vi "Func-엑셀 데이터를 그래프로 출력.vi"() -> ()   [LabVIEW 2015] (continued)
-40\t-40.02\t-26.852\n-40\t-40.02\t-26.858\n-40\t-40\t-26.864\n-40\t-40\t-26.866\n-40\t-40\t-26.87\n-40\t-40\t-26.875\n-40\t-40\t-26.878\n-40\t-40\t-26.884\n-40\t-40\t-26.888\n-40\t-40\t-26.889\n-40\t-40\t-26.893\n-40\t-40\t-26.896\n-40\t-40\t-26.899\n-40\t-40\t-26.902\n-40\t-40\t-26.903\n-40\t-40\t-26.909\n-40\t-40\t-26.915\n-40\t-40\t-26.918\n-40\t-40\t-26.925\n-40\t-40\t-26.93\n-40\t-40\t-26.935\n-40\t-40\t-26.936\n-40\t-40\t-26.938\n-40\t-40\t-26.943\n-40\t-40\t-26.944\n-40\t-40\t-26.948\n-40\t-40\t-26.952\n-40\t-40\t-26.958\n-40\t-40\t-26.965\n-40\t-40\t-26.968\n-40\t-40\t-26.972\n-40\t-40\t-26.973\n-40\t-40\t-26.979\n-40\t-40\t-26.978\n-40\t-40\t-26.982\n-40\t-40\t-26.987\n-40\t-40\t-26.992\n-40\t-40\t-27\n-40\t-40\t-27.002\n-40\t-40\t-27.007\n-40\t-40\t-27.009\n-40\t-40\t-27.012\n-40\t-40\t-27.013\n-40\t-40\t-27.022\n-40\t-40\t-27.022\n-40\t-40\t-27.027\n-40\t-40\t-27.032\n-40\t-40\t-27.035\n-40\t-40\t-27.038\n-40\t-40\t-27.037\n-40\t-40\t-27.04\n-40\t-40\t-27.042\n-40\t-40\t-27.049\n-40\t-40\t-27.05\n-40\t-40\t-27.053\n-40\t-40\t-27.059\n-40\t-40\t-27.064\n-40\t-40\t-27.07\n-40\t-40\t-27.073\n-40\t-40.02\t-27.078\n-40\t-40.02\t-27.08\n-40\t-40.02\t-27.088\n-40\t-40.02\t-27.095\n-40\t-40.02\t-27.096\n-40\t-40.02\t-27.103\n-40\t-40.02\t-27.105\n-40\t-40.02\t-27.11\n-40\t-40.02\t-27.113\n-40\t-40.02\t-27.11\n-40\t-40.02\t-27.114\n-40\t-40.02\t-27.115\n-40\t-40.02\t-27.12\n-40\t-40.02\t-27.123\n-40\t-40.02\t-27.126\n-40\t-40.02\t-27.132\n-40\t-40.02\t-27.136\n-40\t-40.02\t-27.143\n-40\t-40.02\t-27.143\n-40\t-40.02\t-27.145\n-40\t-40.02\t-27.148\n-40\t-40.02\t-27.153\n-40\t-40.02\t-27.157\n-40\t-40.02\t-27.164\n-40\t-40.02\t-27.168\n-40\t-40.02\t-27.173\n-40\t-40.02\t-27.18\n-40\t-40.02\t-27.184\n-40\t-40.02\t-27.186\n-40\t-40.02\t-27.184\n-40\t-40.02\t-27.19\n-40\t-40.02\t-27.194\n-40\t-40.02\t-27.196\n-40\t-40.02\t-27.2\n-40\t-40.02\t-27.202\n-40\t-40.02\t-27.209\n-40\t-40.02\t-27.208\n-40\t-40.02\t-27.211\n-40\t-40.02\t-27.219\n-40\t-40.02\t-27.222\n-40\t-40.02\t-27.227\n-40\t-40.02\t-27.23\n-40\t-40.02\t-27.237\n-40\t-40.02\t-27.241\n-40\t-40.02\t-27.241\n-40\t-40.02\t-27.243\n-40\t-40.02\t-27.248\n-40\t-40.02\t-27.255\n-40\t-40.02\t-27.257\n-40\t-40.02\t-27.259\n-40\t-40.02\t-27.264\n-40\t-40.02\t-27.268\n-40\t-40.02\t-27.27\n-40\t-40.02\t-27.277\n-40\t-40.02\t-27.278\n-40\t-40.02\t-27.279\n-40\t-40.02\t-27.282\n-40\t-40.02\t-27.284\n-40\t-40.02\t-27.285\n-40\t-40.02\t-27.283\n-40\t-40.02\t-27.286\n-40\t-40.02\t-27.293\n-40\t-40.02\t-27.298\n-40\t-40.02\t-27.303\n-40\t-40.02\t-27.308\n-40\t-40.02\t-27.312\n-40\t-40.02\t-27.315\n-40\t-40.02\t-27.318\n-40\t-40.02\t-27.324\n-40\t-40\t-27.327\n-40\t-40\t-27.33\n-40\t-40\t-27.335\n-40\t-40\t-27.342\n-40\t-40\t-27.344\n-40\t-40\t-27.344\n-40\t-40\t-27.349\n-40\t-40\t-27.349\n-40\t-40\t-27.355\n-40\t-40\t-27.356\n-40\t-40\t-27.361\n-40\t-40\t-27.371\n-40\t-40\t-27.373\n-40\t-40\t-27.375\n-40\t-40\t-27.382\n-40\t-40\t-27.385\n-40\t-40\t-27.388\n-40\t-40\t-27.389\n-40\t-40\t-27.393\n-40\t-40\t-27.398\n-40\t-40\t-27.397\n-40\t-40\t-27.398\n-40\t-40\t-27.401\n-40\t-40\t-27.401\n-40\t-40\t-27.404\n-40\t-40\t-27.412\n-40\t-40\t-27.414\n-40\t-40\t-27.417\n-40\t-40\t-27.421\n-40\t-40\t-27.429\n-40\t-40\t-27.431\n-40\t-40\t-27.435\n-40\t-40\t-27.439\n-40\t-40\t-27.444\n-40\t-40\t-27.443\n-40\t-40\t-27.449\n-40\t-40\t-27.451\n-40\t-40\t-27.453\n-40\t-40\t-27.453\n-40\t-40\t-27.453\n-40\t-40\t-27.456\n-40\t-40\t-27.461\n-40\t-40\t-27.461\n-40\t-40\t-27.466\n-40\t-40\t-27.473\n-40\t-40\t-27.477\n-40\t-40\t-27.481\n-40\t-40\t-27.482\n-40\t-40\t-27.488\n-40\t-40\t-27.492\n-40\t-40\t-27.497\n-40\t-40\t-27.502\n-40\t-40\t-27.504\n-40\t-40\t-27.507\n-40\t-40\t-27.507\n-40\t-40\t-27.51\n-40\t-40\t-27.515\n-40\t-40\t-27.516\n-40\t-40\t-27.524\n-40\t-40\t-27.533\n-40\t-40\t-27.538\n-40\t-40\t-27.54\n-40\t-40\t-27.539\n-40\t-40\t-27.543\n-40\t-40\t-27.546\n-40\t-40\t-27.546\n-40\t-40\t-27.548\n-40\t-40\t-27.549\n-40\t-40\t-27.553\n-40\t-40\t-27.557\n-40\t-40\t-27.557\n-40\t-40\t-27.559\n-40\t-40\t-27.562\n-40\t-40\t-27.569\n-40\t-40\t-27.572\n-40\t-40\t-27.571\n-40\t-40\t-27.579\n-40\t-40\t-27.582\n-40\t-40\t-27.586\n-40\t-40\t-27.588\n-40\t-40\t-27.591\n-40\t-40\t-27.594\n-40\t-40\t-27.595\n-40\t-40\t-27.595\n-40\t-40\t-27.599\n-40\t-40\t-27.605\n-40\t-40\t-27.607\n-40\t-40\t-27.61\n-40\t-40\t-27.613\n-40\t-40\t-27.616\n-40\t-40\t-27.619\n-40\t-40\t-27.623\n-40\t-40\t-27.627\n-40\t-40\t-27.634\n-40\t-40\t-27.64\n-40\t-40\t-27.646\n-40\t-40\t-27.647\n-40\t-40\t-27.652\n-40\t-40\t-27.654\n-40\t-40\t-27.654\n-40\t-40\t-27.655\n-40\t-40\t-27.655\n-40\t-40\t-27.658\n-40\t-40\t-27.659\n-40\t-40\t-27.663\n-40\t-40\t-27.668\n-40\t-40\t-27.674\n-40\t-40\t-27.675\n-40\t-40\t-27.678\n-40\t-40\t-27.682\n-40\t-40\t-27.687\n-40\t-40\t-27.686\n-40\t-40\t-27.689\n-40\t-40\t-27.695\n-40\t-40\t-27.698\n-40\t-40\t-27.703\n-40\t-40\t-27.705\n-40\t-40\t-27.707\n-40\t-40\t-27.712\n-40\t-40\t-27.714\n-40\t-40\t-27.715\n-40\t-40\t-27.719\n-40\t-40\t-27.721\n-40\t-40\t-27.726\n-40\t-40\t-27.729\n-40\t-40\t-27.732\n-40\t-40\t-27.734\n-40\t-40\t-27.735\n-40\t-40\t-27.734\n-40\t-40\t-27.738\n-40\t-40\t-27.739\n-40\t-40\t-27.741\n-40\t-40\t-27.746\n-40\t-40\t-27.753\n-40\t-40\t-27.758\n-40\t-40\t-27.762\n-40\t-40\t-27.762\n-40\t-40\t-27.765\n-40\t-40\t-27.769\n-40\t-40\t-27.768\n-40\t-40\t-27.769\n-40\t-40\t-27.77\n-40\t-40\t-27.777\n-40\t-40\t-27.781\n-40\t-40\t-27.781\n-40\t-40\t-27.788\n-40\t-40\t-27.793\n-40\t-40\t-27.796\n-40\t-40\t-27.8\n-40\t-40\t-27.804\n-40\t-40\t-27.807\n-40\t-40\t-27.809\n-40\t-40\t-27.81\n-40\t-40\t-27.811\n-40\t-40\t-27.815\n-40\t-40\t-27.814\n-40\t-40\t-27.816\n-40\t-40\t-27.821\n-40\t-40\t-27.825\n-40\t-40\t-27.827\n-40\t-40\t-27.831\n-40\t-40\t-27.835\n-40\t-40\t-27.837\n-40\t-40\t-27.841\n-40\t-40\t-27.843\n-40\t-40\t-27.846\n-40\t-40\t-27.85\n-40\t-40\t-27.854\n-40\t-40\t-27.858\n-40\t-40\t-27.862\n-40\t-40\t-27.864\n-40\t-40\t-27.868\n-40\t-40\t-27.871\n-40\t-40\t-27.877\n-40\t-40\t-27.878\n-40\t-40\t-27.88\n-40\t-40\t-27.883\n-40\t-40\t-27.884\n-40\t-40\t-27.885\n-40\t-40\t-27.885\n-40\t-40\t-27.888\n-40\t-40\t-27.889\n-40\t-40\t-27.891\n-40\t-40\t-27.895\n-40\t-40\t-27.902\n-40\t-40\t-27.903\n-40\t-40\t-27.905\n-40\t-40\t-27.908\n-40\t-40\t-27.909\n-40\t-40\t-27.914\n-40\t-40\t-27.914\n-40\t-40\t-27.918\n-40\t-40\t-27.918\n-40\t-40\t-27.921\n-40\t-40\t-27.927\n-40\t-40\t-27.927\n-40\t-40\t-27.933\n-40\t-40\t-27.936\n-40\t-40\t-27.939\n-40\t-40\t-27.943\n-40\t-40\t-27.943\n-40\t-40\t-27.949\n-40\t-40\t-27.955\n-40\t-40\t-27.957\n-40\t-40\t-27.962\n-40\t-40\t-27.966\n-40\t-40\t-27.966\n-40\t-40\t-27.963\n-40\t-40\t-27.963\n-40\t-40\t-27.966\n-40\t-40\t-27.968\n-40\t-40\t-27.971\n-40\t-40\t-27.975\n-40\t-40\t-27.979\n-40\t-40\t-27.981\n-40\t-40\t-27.982\n-40\t-40\t-27.983\n-40\t-40\t-27.98\n-40\t-40\t-27.983\n-40\t-40\t-27.984\n-40\t-40\t-27.989\n-40\t-40\t-27.991\n-40\t-40\t-27.997\n-40\t-40\t-28.002\n-40\t-40\t-28.004\n-40\t-40\t-28.005\n-40\t-40\t-28.006\n-40\t-40\t-28.013\n-40\t-40\t-28.016\n-40\t-40\t-28.018\n-40\t-40\t-28.021\n-40\t-40\t-28.029\n-40\t-40\t-28.032\n-40\t-40\t-28.031\n-40\t-40\t-28.034\n-40\t-40\t-28.037\n-40\t-40\t-28.043\n-40\t-40\t-28.045\n-40\t-40\t-28.045\n-40\t-40\t-28.048\n-40\t-40\t-28.049\n-40\t-40\t-28.052\n-40\t-40\t-28.055\n-40\t-40\t-28.062\n-40\t-40\t-28.065\n-40\t-40\t-28.067\n-40\t-40\t-28.074\n-40\t-40\t-28.076\n-40\t-40\t-28.075\n-40\t-40\t-28.076\n-40\t-40\t-28.078\n-40\t-40\t-28.077\n-40\t-40\t-28.081\n-40\t-40\t-28.087\n-40\t-40\t-28.087\n-40\t-40\t-28.09\n-40\t-40\t-28.095\n-40\t-40\t-28.102\n-40\t-40\t-28.103\n-40\t-40\t-28.102\n-40\t-40\t-28.104\n-40\t-40\t-28.108\n-40\t-40\t-28.108\n-40\t-40\t-28.108\n-40\t-40\t-28.108\n-40\t-40\t-28.111\n-40\t-40\t-28.117\n-40\t-40\t-28.117\n-40\t-40\t-28.119\n-40\t-40\t-28.121\n-40\t-40\t-28.125\n-40\t-40\t-28.125\n-40\t-40\t-28.127\n-40\t-40\t-28.129\n-40\t-40\t-28.134\n-40\t-40\t-28.135\n-40\t-40\t-28.139\n-40\t-40\t-28.141\n-40\t-40\t-28.143\n-40\t-40\t-28.149\n-40\t-40\t-28.153\n-40\t-40\t-28.155\n-40\t-40\t-28.157\n-40\t-40\t-28.16\n-40\t-40\t-28.164\n-40\t-40\t-28.165\n-40\t-40\t-28.17\n-40\t-40\t-28.175\n-40\t-40\t-28.18\n-40\t-40\t-28.183\n-40\t-40\t-28.182\n-40\t-40\t-28.186\n-40\t-40\t-28.182\n-40\t-40\t-28.182\n-40\t-40\t-28.184\n-40\t-40\t-28.184\n-40\t-40\t-28.19\n-40\t-40\t-28.194\n-40\t-40\t-28.198\n-40\t-40\t-28.203\n-40\t-40\t-28.205\n-40\t-40\t-28.208\n-40\t-40\t-28.209\n-40\t-40\t-28.21\n-40\t-40\t-28.212\n-40\t-40\t-28.212\n-40\t-40\t-28.217\n-40\t-40\t-28.221\n-40\t-40\t-28.223\n-40\t-40\t-28.225\n-40\t-40\t-28.223\n-40\t-40\t-28.228\n-40\t-40\t-28.23\n-40\t-40\t-28.233\n-40\t-40\t-28.233\n-40\t-40\t-28.236\n-40\t-40\t-28.239\n-40\t-40\t-28.237\n-40\t-40\t-28.239\n-40\t-40\t-28.24\n-40\t-40\t-28.244\n-40\t-40\t-28.245\n-40\t-40\t-28.25\n-40\t-40\t-28.255\n-40\t-40\t-28.258\n-40\t-40\t-28.259\n-40\t-40\t-28.261\n-40\t-40\t-28.263\n-40\t-40\t-28.265\n-40\t-40\t-28.264\n-40\t-40\t-28.261\n-40\t-40\t-28.263\n-40\t-40\t-28.269\n-40\t-40\t-28.273\n-40\t-40\t-28.273\n-40\t-40\t-28.277\n-40\t-40\t-28.284\n-40\t-40\t-28.29\n-40\t-40\t-28.288\n-40\t-40\t-28.291\n-40\t-40\t-28.295\n-40\t-40\t-28.298\n-40\t-40\t-28.3\n-40\t-40\t-28.298\n-40\t-40\t-28.302\n-40\t-40\t-28.307\n-40\t-40\t-28.308\n-40\t-40\t-28.313\n-40\t-40\t-28.314\n-40\t-40\t-28.318\n-40\t-40\t-28.321\n-40\t-40\t-28.319\n-40\t-40\t-28.322\n-40\t-40\t-28.318\n-40\t-40\t-28.322\n-40\t-40\t-28.324\n-40\t-40\t-28.323\n-40\t-40\t-28.329\n-40\t-40\t-28.334\n-40\t-40\t-28.337\n-40\t-40\t-28.343\n-40\t-40\t-28.343\n-40\t-40\t-28.347\n-40\t-40\t-28.351\n-40\t-40\t-28.348\n-40\t-40\t-28.352\n-40\t-40\t-28.354\n-40\t-40\t-28.355\n-40\t-40\t-28.356\n-40\t-40\t-28.355\n-40\t-40\t-28.36\n-40\t-40\t-28.36\n-40\t-40\t-28.357\n-40\t-40\t-28.362\n-40\t-40\t-28.365\n-40\t-40\t-28.369\n-40\t-40\t-28.371\n-40\t-40\t-28.373\n-40\t-40\t-28.38\n-40\t-40\t-28.381\n-40\t-40\t-28.384\n-40\t-40\t-28.384\n-40\t-40\t-28.388\n-40\t-40\t-28.391\n-40\t-40\t-28.391\n-40\t-40\t-28.391\n-40\t-40\t-28.394\n-40\t-40\t-28.395\n-40\t-40\t-28.394\n-40\t-40\t-28.398\n-40\t-40\t-28.403\n-40\t-40\t-28.404\n-40\t-40\t-28.406\n-40\t-40\t-28.409\n-40\t-40\t-28.413\n-40\t-40\t-28.411\n-40\t-40\t-28.411\n-40\t-40\t-28.412\n-40\t-40\t-28.417\n-40\t-40\t-28.418\n-40\t-40\t-28.42\n-40\t-40\t-28.425\n-40\t-40\t-28.43\n-40\t-40\t-28.434\n-40\t-40\t-28.435\n-40\t-40\t-28.436\n-40\t-40\t-28.436\n-40\t-40\t-28.44\n-40\t-40\t-28.44\n-40\t-40\t-28.445\n-40\t-40\t-28.446\n-40\t-40\t-28.449\n-40\t-40\t-28.451\n-40\t-40\t-28.449\n-40\t-40\t-28.45\n-40\t-40\t-28.45\n-40\t-40\t-28.452\n-40\t-40\t-28.451\n-40\t-40\t-28.457\n-40\t-40\t-28.46\n-40\t-40\t-28.46\n-40\t-40\t-28.459\n-40\t-40\t-28.464\n-40\t-40\t-28.469\n-40\t-40\t-28.467\n-40\t-40\t-28.471\n-40\t-40\t-28.474\n-40\t-40\t-28.479\n-40\t-40\t-28.478\n-40\t-40\t-28.478\n-40\t-40.02\t-28.479\n-40\t-40.02\t-28.481\n-40\t-40.02\t-28.486\n-40\t-40\t-28.489\n-40\t-40.02\t-28.49\n-40\t-40\t-28.491\n-40\t-40\t-28.493\n-40\t-40\t-28.492\n-40\t-40\t-28.492\n-40\t-40\t-28.488\n-40\t-40\t-28.497\n-40\t-40\t-28.503\n-40\t-40\t-28.502\n-40\t-40\t-28.507\n-40\t-40\t-28.513\n-40\t-40.02\t-28.519\n-40\t-40.02\t-28.517\n-40\t-40.02\t-28.516\n-40\t-40.02\t-28.522\n-40\t-40.02\t-28.526\n-40\t-40\t-28.524\n-40\t-40\t-28.527\n-40\t-40\t-28.534\n-40\t-40\t-28.535\n-40\t-40.02\t-28.536\n-40\t-40.02\t-28.538\n-40\t-40.02\t-28.54\n-40\t-40.02\t-28.539\n-40\t-40.02\t-28.539\n-40\t-40.02\t-28.54\n-40\t-40.02\t-28.543\n-40\t-40.02\t-28.546\n-40\t-40.02\t-28.547\n-40\t-40.02\t-28.549\n-40\t-40.02\t-28.549\n-40\t-40.02\t-28.553\n-40\t-40.02\t-28.554\n-40\t-40.02\t-28.555\n-40\t-40.02\t-28.559\n-40\t-40.02\t-28.564\n-40\t-40.02\t-28.565\n-40\t-40\t-28.564\n-40\t-40\t-28.565\n-40\t-40\t-28.567\n-40\t-40\t-28.567\n-40\t-40\t-28.565\n-40\t-40\t-28.566\n-40\t-40\t-28.569\n-40\t-40\t-28.57\n-40\t-40\t-28.574\n-40\t-40.02\t-28.577\n-40\t-40\t-28.579\n-40\t-40\t-28.584\n-40\t-40\t-28.586\n-40\t-40\t-28.589\n-40\t-40\t-28.59\n-40\t-40\t-28.589\n-40\t-40\t-28.591\n-40\t-40\t-28.594\n-40\t-40\t-28.595\n-40\t-40\t-28.595\n-40\t-40\t-28.598\n-40\t-40\t-28.599\n-40\t-40\t-28.601\n-40\t-40\t-28.607\n-40\t-40\t-28.609\n-40\t-40\t-28.609\n-40\t-40\t-28.613\n-40\t-40\t-28.615\n-40\t-40\t-28.616\n-40\t-40\t-28.613\n-40\t-40\t-28.615\n-40\t-40\t-28.619\n-40\t-40\t-28.618\n-40\t-40\t-28.621\n-40\t-40\t-28.623\n-40\t-40.02\t-28.626\n-40\t-40\t-28.628\n-40\t-40\t-28.632\n-40\t-40\t-28.635\n-40\t-40\t-28.636\n-40\t-40\t-28.639\n-40\t-40\t-28.638\n-40\t-40\t-28.639\n-40\t-40\t-28.639\n-40\t-40\t-28.64\n-40\t-40\t-28.641\n-40\t-40\t-28.643\n-40\t-40\t-28.649\n-40\t-40\t-28.651\n-40\t-40\t-28.65\n-40\t-40\t-28.654\n-40\t-40\t-28.655\n-40\t-40\t-28.656\n-40\t-40\t-28.658\n-40\t-40\t-28.659\n-40\t-40\t-28.659\n-40\t-40\t-28.661\n-40\t-40\t-28.664\n-40\t-40\t-28.666\n-40\t-40\t-28.668\n-40\t-40\t-28.671\n-40\t-40\t-28.673\n-40\t-40\t-28.679\n-40\t-40\t-28.68\n-40\t-40\t-28.682\n-40\t-40\t-28.683\n-40\t-40\t-28.684\n-40\t-40\t-28.69\n-40\t-40\t-28.69\n-40\t-40\t-28.69\n-40\t-40\t-28.696\n-40\t-40\t-28.7\n-40\t-40\t-28.702\n-40\t-40\t-28.701\n-40\t-40\t-28.703\n-40\t-40\t-28.706\n-40\t-40\t-28.706\n-40\t-40\t-28.703\n-40\t-40\t-28.704\n-40\t-40\t-28.707\n-40\t-40\t-28.71\n-40\t-40\t-28.71\n-40\t-40\t-28.71\n-40\t-40\t-28.712\n-40\t-40\t-28.712\n-40\t-40\t-28.712\n-40\t-40\t-28.71\n-40\t-40\t-28.714\n-40\t-40\t-28.717\n-40\t-40\t-28.719\n-40\t-40\t-28.721\n-40\t-40\t-28.726\n-40\t-40\t-28.727\n-40\t-40\t-28.728\n-40\t-40\t-28.731\n-40\t-40\t-28.736\n-40\t-40\t-28.736\n-40\t-40\t-28.734\n-40\t-40\t-28.739\n-40\t-40\t-28.741\n-40\t-40\t-28.741\n-40\t-40\t-28.739\n-40\t-40\t-28.74\n-40\t-40\t-28.743\n-40\t-40\t-28.746\n-40\t-40\t-28.747\n-40\t-40\t-28.746\n-40\t-40\t-28.751\n-40\t-40\t-28.754\n-40\t-40\t-28.755\n-40\t-40\t-28.761\n-40\t-40\t-28.762\n-40\t-40\t-28.762\n-40\t-40\t-28.761\n-40\t-40\t-28.763\n-40\t-40\t-28.764\n-40\t-40\t-28.764\n-40\t-40\t-28.765\n-40\t-40\t-28.773\n-40\t-40\t-28.775\n-40\t-40\t-28.777\n-40\t-40\t-28.783\n-40\t-40\t-28.779\n-40\t-40\t-28.782\n-40\t-40\t-28.781\n-40\t-40\t-28.783\n-40\t-40\t-28.783\n-40\t-40\t-28.782\n-40\t-40\t-28.786\n-40\t-40\t-28.786\n-40\t-40\t-28.79\n-40\t-40\t-28.79\n-40\t-40\t-28.791\n-40\t-40\t-28.798\n-40\t-40\t-28.799\n-40\t-40\t-28.8\n-40\t-40\t-28.801\n-40\t-40\t-28.802\n-40\t-40\t-28.804\n-40\t-40\t-28.804\n-40\t-40\t-28.807\n-40\t-40\t-28.805\n-40\t-40\t-28.809\n-40\t-40\t-28.811\n-40\t-40\t-28.811\n-40\t-40\t-28.814\n-40\t-40\t-28.812\n-40\t-40\t-28.819\n-40\t-40\t-28.821\n-40\t-40\t-28.821\n-40\t-40\t-28.824\n-40\t-40\t-28.825\n-40\t-40\t-28.83\n-40\t-40\t-28.825\n-40\t-40\t-28.829\n-40\t-40\t-28.833\n-40\t-40\t-28.834\n-40\t-40\t-28.834\n-40\t-40\t-28.832\n-40\t-40\t-28.836\n-40\t-40\t-28.834\n-40\t-40\t-28.838\n-40\t-40\t-28.841\n-40\t-40\t-28.844\n-40\t-40\t-28.847\n-40\t-40\t-28.85\n-40\t-40\t-28.851\n-40\t-40\t-28.851\n-40\t-40\t-28.852\n-40\t-40\t-28.852\n-40\t-40\t-28.852\n-40\t-40\t-28.855\n-40\t-40\t-28.86\n-40\t-40\t-28.863\n-40\t-40\t-28.866\n-40\t-40\t-28.869\n-40\t-40\t-28.871\n-40\t-40\t-28.872\n-40\t-40\t-28.872\n-40\t-40\t-28.871\n-40\t-40\t-28.872\n-40\t-40\t-28.873\n-40\t-40\t-28.873\n-40\t-40\t-28.873\n-40\t-40\t-28.874\n-40\t-40\t-28.875\n-40\t-40\t-28.875\n-40\t-40\t-28.879\n-40\t-40\t-28.885\n-40\t-40\t-28.884\n-40\t-40\t-28.886\n-40\t-40\t-28.891\n-40\t-40\t-28.893\n-40\t-40\t-28.893\n-40\t-40\t-28.891\n-40\t-40\t-28.893\n-40\t-40\t-28.896\n-40\t-40\t-28.895\n-40\t-40\t-28.898\n-40\t-40\t-28.9\n-40\t-40\t-28.9\n-40\t-40\t-28.902\n-40\t-40\t-28.904\n-40\t-40\t-28.906\n-40\t-40\t-28.907\n-40\t-40\t-28.908\n-40\t-40\t-28.909\n-40\t-40\t-28.908\n-40\t-40\t-28.911\n-40\t-40\t-28.911\n-40\t-40\t-28.914\n-40\t-40\t-28.913\n-40\t-40\t-28.916\n-40\t-40\t-28.917\n-40\t-40\t-28.915\n-40\t-40\t-28.915\n-40\t-40\t-28.913\n-40\t-40\t-28.914\n-40\t-40\t-28.916\n-40\t-40\t-28.92\n-40\t-40\t-28.924\n-40\t-40\t-28.923\n-40\t-40\t-28.923\n-40\t-40\t-28.928\n-40\t-40\t-28.93\n-40\t-40.02\t-28.931\n-40\t-40.02\t-28.931\n-40\t-40.02\t-28.934\n-40\t-40.02\t-28.935\n-40\t-40.02\t-28.937\n-40\t-40.02\t-28.935\n-40\t-40.02\t-28.937\n-40\t-40.02\t-28.94\n-40\t-40\t-28.942\n-40\t-40\t-28.948\n-40\t-40\t-28.95\n-40\t-40\t-28.954\n-40\t-40\t-28.956\n-40\t-40\t-28.957\n-40\t-40\t-28.955\n-40\t-40\t-28.954\n-40\t-40\t-28.954\n-40\t-40\t-28.954\n-40\t-40\t-28.953\n-40\t-40\t-28.956\n-40\t-40\t-28.962\n-40\t-40\t-28.961\n-40\t-40\t-28.966\n-40\t-40\t-28.968\n-40\t-40\t-28.971\n-40\t-40\t-28.973\n-40\t-40\t-28.973\n-40\t-40\t-28.975\n-40\t-40\t-28.975\n-40\t-40\t-28.979\n-40\t-40\t-28.98\n-40\t-40\t-28.982\n-40\t-40\t-28.983\n-40\t-40\t-28.986\n-40\t-40\t-28.989\n-40\t-40\t-28.989\n-40\t-40\t-28.989\n-40\t-40\t-28.995\n-40\t-40\t-28.997\n-40\t-40\t-28.998\n-40\t-40\t-28.999\n-40\t-40\t-29\n-40\t-40\t-28.999\n-40\t-40\t-28.998\n-40\t-40\t-28.999\n-40\t-40\t-29.001\n-40\t-40\t-29.001\n-40\t-40\t-29\n-40\t-40\t-29.004\n-40\t-40\t-29.004\n-40\t-40\t-29.007\n-40\t-40\t-29.011\n-40\t-40\t-29.011\n-40\t-40\t-29.013\n-40\t-40\t-29.013\n-40\t-40\t-29.018\n-40\t-40\t-29.018\n-40\t-40\t-29.016\n-40\t-40\t-29.017\n-40\t-40\t-29.014\n-40\t-40\t-29.018\n-40\t-40\t-29.015\n-40\t-40\t-29.016\n-40\t-40\t-29.017\n-40\t-40\t-29.023\n-40\t-40\t-29.025\n-40\t-40\t-29.023\n-40\t-40\t-29.024\n-40\t-40\t-29.025\n-40\t-40\t-29.024\n-40\t-40\t-29.021\n-40\t-40\t-29.025\n-40\t-40\t-29.026\n-40\t-40\t-29.029\n-40\t-40\t-29.032\n-40\t-40\t-29.036\n-40\t-40\t-29.037\n-40\t-40\t-29.039\n-40\t-40\t-29.041\n-40\t-40\t-29.046\n-40\t-40\t-29.046\n-40\t-40\t-29.048\n-40\t-40\t-29.051\n-40\t-40\t-29.049\n-40\t-40\t-29.048\n-40\t-40\t-29.047\n-40\t-40\t-29.047\n-40\t-40\t-29.047\n-40\t-40\t-29.05\n-40\t-40\t-29.055\n-40\t-40\t-29.06\n-40\t-40\t-29.062\n-40\t-40\t-29.065\n-40\t-40\t-29.069\n-40\t-40.02\t-29.071\n-40\t-40\t-29.068\n-40\t-40\t-29.068\n-40\t-40\t-29.071\n-40\t-40\t-29.07\n-40\t-40\t-29.066\n-40\t-40\t-29.065\n-40\t-40.02\t-29.065\n-40\t-40.02\t-29.065\n-40\t-40.02\t-29.067\n-40\t-40.02\t-29.067\n-40\t-40.02\t-29.071\n-40\t-40.02\t-29.074\n-40\t-40.02\t-29.077\n-40\t-40.02\t-29.079\n-40\t-40.02\t-29.081\n-40\t-40\t-29.086\n-40\t-40\t-29.086\n-40\t-40\t-29.09\n-40\t-40\t-29.091\n-40\t-40\t-29.093\n-40\t-40\t-29.092\n-40\t-40\t-29.092\n-40\t-40\t-29.093\n-40\t-40\t-29.095\n-40\t-40\t-29.094\n-40\t-40\t-29.095\n-40\t-40\t-29.096\n-40\t-40\t-29.098\n-40\t-40\t-29.098\n-40\t-40\t-29.101\n-40\t-40\t-29.102\n-40\t-40\t-29.1\n-40\t-40\t-29.102\n-40\t-40\t-29.101\n-40\t-40\t-29.102\n-40\t-40\t-29.102\n-40\t-40\t-29.105\n-40\t-40\t-29.109\n-40\t-40\t-29.11\n-40\t-40\t-29.111\n-40\t-40\t-29.11\n-40\t-40\t-29.113\n-40\t-40\t-29.113\n-40\t-40\t-29.115\n-40\t-40\t-29.117\n-40\t-40\t-29.116\n-40\t-40\t-29.12\n-40\t-40\t-29.121\n-40\t-40\t-29.122\n-40\t-40\t-29.123\n-40\t-40\t-29.125\n-40\t-40\t-29.125\n-40\t-40\t-29.124\n-40\t-40\t-29.125\n-40\t-40\t-29.125\n-40\t-40\t-29.127\n-40\t-40\t-29.127\n-40\t-40\t-29.13\n-40\t-40\t-29.132\n-40\t-40\t-29.134\n-40\t-40\t-29.137\n-40\t-40\t-29.138\n-40\t-40\t-29.138\n-40\t-40\t-29.141\n-40\t-40\t-29.144\n-40\t-40\t-29.145\n-40\t-40\t-29.146\n-40\t-40\t-29.145\n-40\t-40\t-29.148\n-40\t-40\t-29.148\n-40\t-40\t-29.148\n-40\t-40.02\t-29.152\n-40\t-40.02\t-29.154\n-40\t-40.02\t-29.155\n-40\t-40\t-29.157\n-40\t-40.02\t-29.158\n-40\t-40\t-29.159\n-40\t-40\t-29.154\n-40\t-40\t-29.153\n-40\t-40\t-29.153\n-40\t-40\t-29.152\n-40\t-40\t-29.153\n-40\t-40\t-29.154\n-40\t-40\t-29.159\n-40\t-40\t-29.164\n-40\t-40\t-29.165\n-40\t-40\t-29.167\n-40\t-40\t-29.169\n-40\t-40\t-29.171\n-40\t-40\t-29.175\n-40\t-40\t-29.172\n-40\t-40\t-29.176\n-40\t-40\t-29.181\n-40\t-40\t-29.184\n-40\t-40\t-29.182\n-40\t-40.02\t-29.182\n-40\t-40\t-29.184\n-40\t-40\t-29.184\n-40\t-40\t-29.185\n-40\t-40\t-29.183\n-40\t-40\t-29.185\n-40\t-40\t-29.186\n-40\t-40\t-29.188\n-40\t-40\t-29.187\n-40\t-40\t-29.189\n-40\t-40\t-29.19\n-40\t-40\t-29.189\n-40\t-40\t-29.19\n-40\t-40\t-29.192\n-40\t-40\t-29.195\n-40\t-40\t-29.196\n-40\t-40\t-29.197\n-40\t-40\t-29.201\n-40\t-40\t-29.202\n-40\t-40\t-29.202\n-40\t-40\t-29.203\n-40\t-40\t-29.205\n-40\t-40\t-29.205\n-40\t-40\t-29.207\n-40\t-40\t-29.209\n
